vi "LensAndCameraCalibration-GFV.vi"(8 "error in (no error)":errorcluster, 10 "Variant In":variant, 11 "LensCalibrationCtl":T1=enum."Get Calibration") -> (0 "error out":errorcluster, 3 "Variant Out":variant)   [LabVIEW 2013]
doc: "Use this template to build a VI to use as a subVI."
uses:
  LensCalibrationCtlGFV.ctl
  LensCalibrationModel.ctl
  <vilib>/Utility/file.llb/Read From Spreadsheet File (string).vi
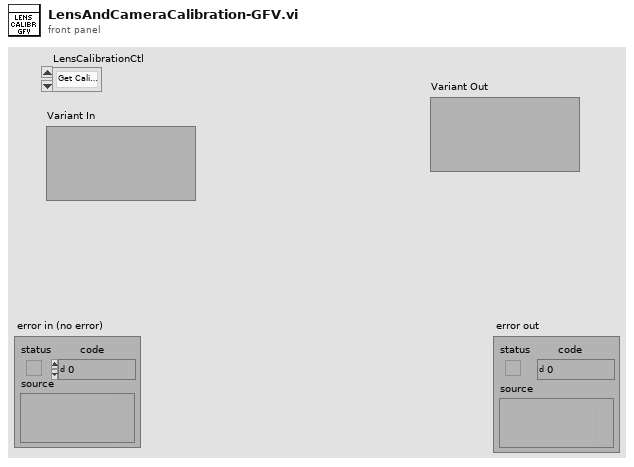
[diagram p1: front panel]
types:
  T1 = typedef "LensCalibrationCtlGFV.ctl" = enum16{"Get MicronPerPixel", "Get Range and PixelsForRange", "Get Mag Names", "Get Calibration", "Read Calibration From File", "Init"}
  T2 = cluster{"MagRingText":u16, "High Resolution":bool}
  T3 = typedef "LensCalibrationModel.ctl" = cluster{"Lens Mag":string, "MicronsPerPixels":dbl, "Scale in microns":i32, "High Resolution":bool}[]
  T4 = cluster{"Lens Mag":string, "MicronsPerPixels":dbl, "Scale in microns":i32, "High Resolution":bool}
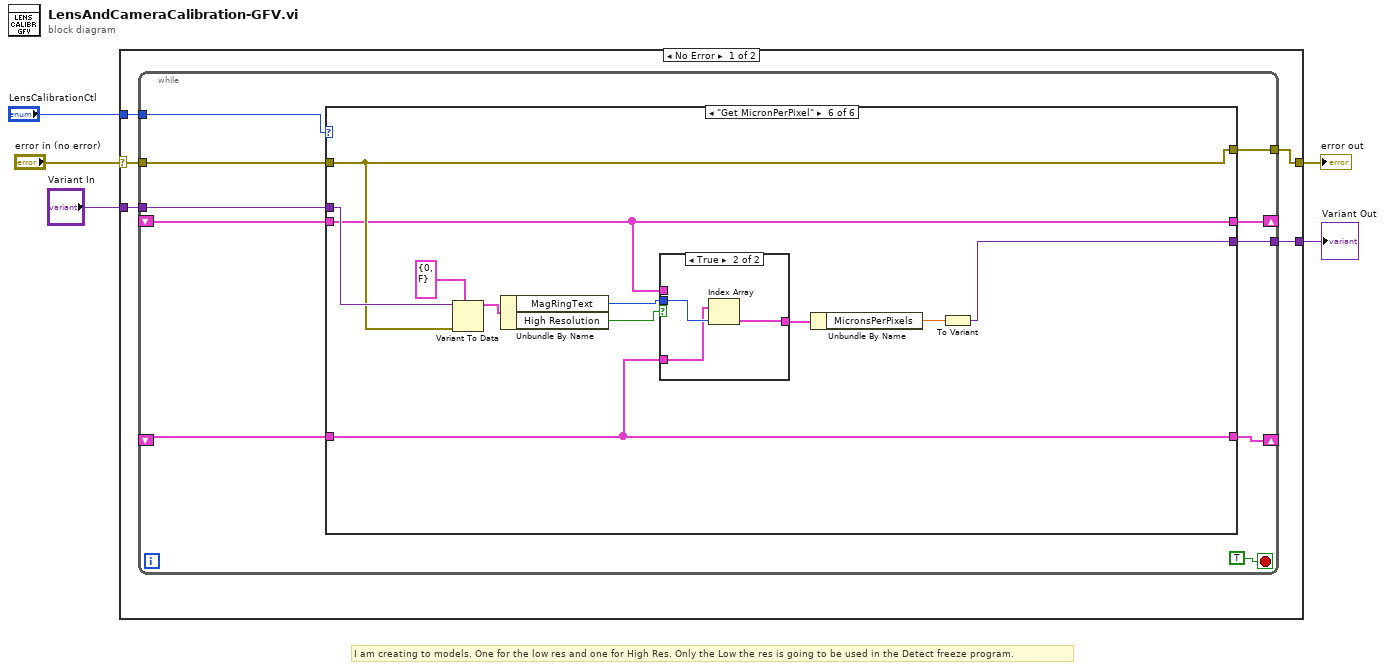
[diagram p0: block diagram]
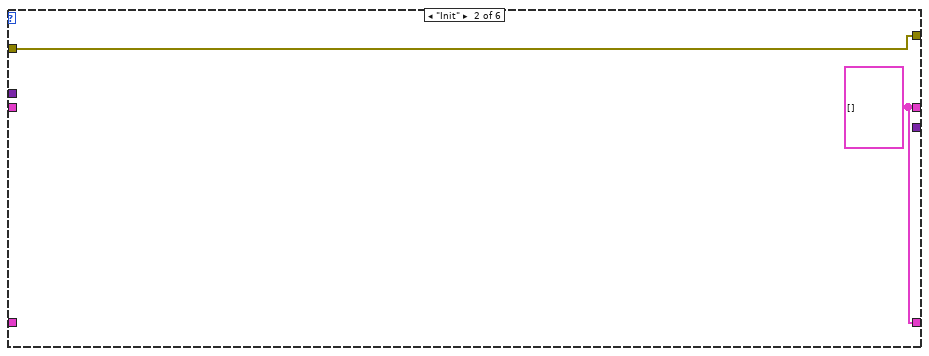
[diagram p3: hidden frame]
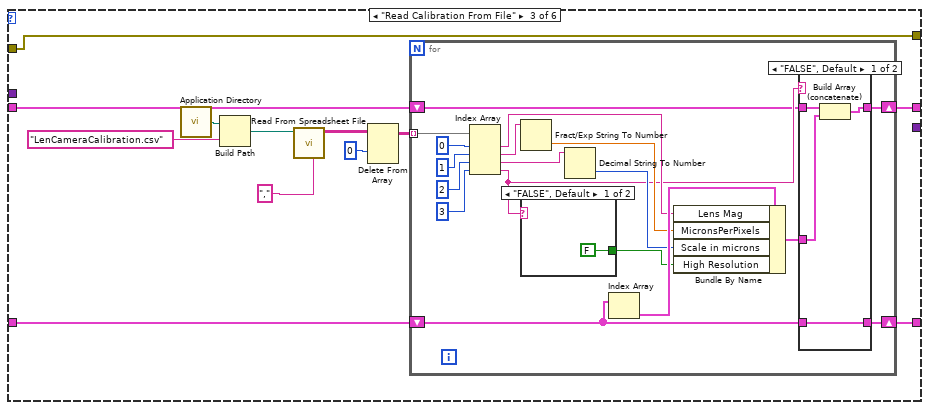
[diagram p4: hidden frame]
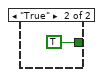
[diagram p5: hidden frame]
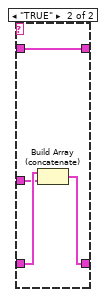
[diagram p6: hidden frame]
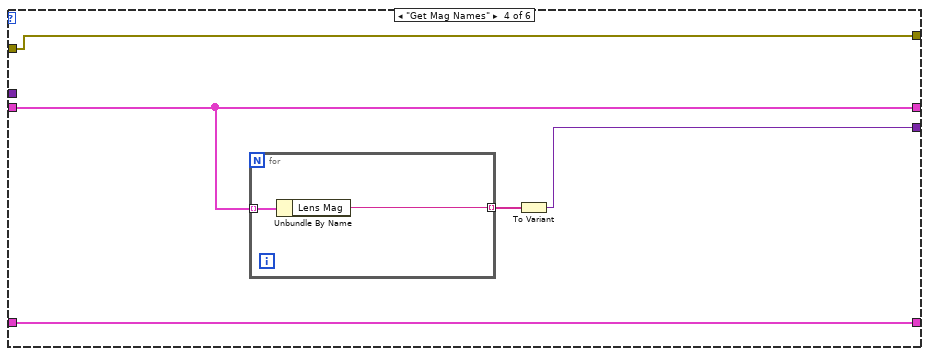
[diagram p7: hidden frame]
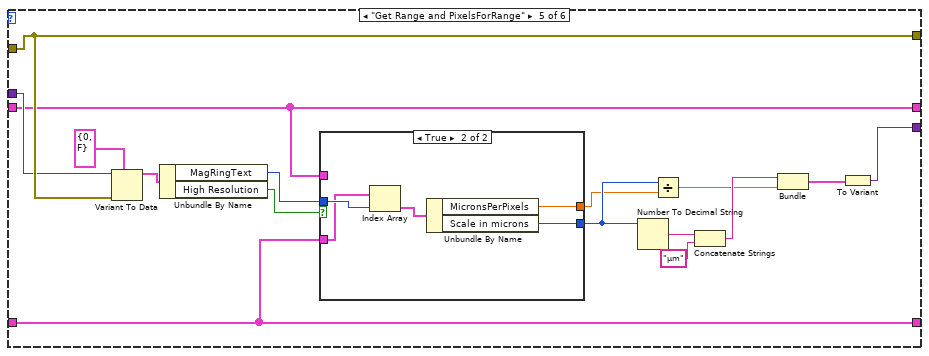
[diagram p8: hidden frame]
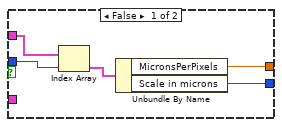
[diagram p9: hidden frame]
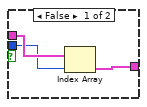
[diagram p10: hidden frame]
diagram:
  # "I am creating to models. One for the low res and one for High Res. Only the Low the res is going to be used in the Detect freeze program."
  n1 = case shown="No Error" "error in (no error)" {
    selector: "error in (no error)" -> [w9 w116]
    tunnel: [w8 w116] -> w4
    tunnel: "LensCalibrationCtl" -> [w10 _]
    tunnel: [w7 _] -> w2
    tunnel: "Variant In" -> [w6 _]
    frame No Error {
      n2 = while {
        tunnel: w10 -> [w19]
        tunnel: w9 -> [w18]
        shift-right: [w14] -> _
        shift-left: _ -> [w15]
        shift-right: [w16] -> _
        shift-left: _ -> [w17]
        tunnel: [w13] -> w8
        tunnel: [w12] -> w7
        tunnel: w6 -> [w11]
        stop <- TRUE stop-if-true
        n3 = case shown="\"Get MicronPerPixel\"" w19 {
          tunnel: w18 -> [w21 w24 w26 w69 w87 w106]
          tunnel: w17 -> [w23 _ w30 w70 w83 w104]
          tunnel: [w23 w25 w29 w70 w83 w104] -> w16
          tunnel: w15 -> [w22 _ w28 w68 w82 w105]
          tunnel: [w22 w25 w27 w68 w82 w105] -> w14
          tunnel: [w21 w24 w26 w69 w87 w106] -> w13
          tunnel: [_ _ _ w66 w77 w99] -> w12
          tunnel: w11 -> [_ _ _ _ w86 w107]
          frame "Get Calibration", Default {
          }
          frame "Init" {
            w25 = T3 [] ("LensLowRes")
          }
          frame "Read Calibration From File" {
            n4 = call <vilib>:"Application Directory.vi"() -> ("Application Directory"=w34:path)
            n5 = Build Path(base path=w34, name or relative path="LenCameraCalibration.csv") -> (appended path=w32:path)
            n6 = call-poly <vilib>:"Read From Spreadsheet File.vi"("delimiter (\\t)"="," ("delimiter (\\t)"), "file path (dialog if empty)"=w32) -> ("all rows"=w36:string[][])  [unwired: 5 in, 4 out]
            n7 = Delete From Array(array=w36, index (row)=0 ("index")) -> (array with subset deleted=w37:string[][])  [unwired: 2 in, 1 out]
            n8 = for {
              tunnel: w37 -> [w55] mode=indexing
              shift-right: [w38] -> w27
              shift-left: w28 -> [w39]
              shift-right: [w45] -> w29
              shift-left: w30 -> [w47]
              n9 = Index Array(array=w55, index #1=0 ("index"), index #2=1 ("index"), index #3=2 ("index"), index #4=3 ("index")) -> (element #1=w44:string, element #2=w50:string, element #3=w49:string, element #4=w41:string)
              n10 = Fract/Exp String To Number(string=w50) -> (number=w43:dbl)  [unwired: 3 in, 1 out]
              n11 = case shown="\"FALSE\", Default" w41 {
                tunnel: [FALSE TRUE] -> w40
                frame "FALSE", Default {
                }
                frame "True" {
                }
              }
              n12 = Decimal String To Number(string=w49) -> (number=w42:i32)  [unwired: 2 in, 1 out]
              n13 = Index Array(array=w47) -> (element=w48:T4)  [unwired: 1 in]
              n14 = Bundle By Name(cluster=w48, "Lens Mag"=w44, "MicronsPerPixels"=w43, "Scale in microns"=w42, "High Resolution"=w40) -> (w46:T4)
              n15 = case shown="\"FALSE\", Default" w41 {
                tunnel: w47 -> [w58 w65]
                tunnel: w46 -> [w60 w64]
                tunnel: [w58 w63] -> w45
                tunnel: w39 -> [w61 w62]
                tunnel: [w59 w62] -> w38
                frame "FALSE", Default {
                  n16 = Build Array (concatenate)(w61, w60) -> (w59:T3)
                }
                frame "TRUE" {
                  n17 = Build Array (concatenate)(w65, w64) -> (w63:T3)
                }
              }
            }
          }
          frame "Get Mag Names" {
            n18 = for {
              tunnel: w68 -> [w72] mode=indexing
              tunnel: [w71] -> w67 mode=indexing
              n19 = Unbundle By Name(w72) -> ("Lens Mag"=w71:string)
            }
            n20 = To Variant(anything=w67) -> (Variant=w66:variant)
          }
          frame "Get Range and PixelsForRange" {
            n21 = Variant To Data(error in=w87, type=T2 {"MagRingText"=0, "High Resolution"=FALSE} ("output cluster"), Variant=w86) -> (data=w85:T2)  [unwired: 1 out]
            n22 = Unbundle By Name(w85) -> ("MagRingText"=w81:u16, "High Resolution"=w84:bool)
            n23 = case shown="True" w84 {
              tunnel: w83 -> [_ w94]
              tunnel: w82 -> [w92 _]
              tunnel: w81 -> [w93 w98]
              tunnel: [w90 w96] -> w74
              tunnel: [w89 w95] -> w75
              frame False {
                n24 = Index Array(array=w92, index=w93) -> (element=w91:T4)
                n25 = Unbundle By Name(w91) -> ("MicronsPerPixels"=w90:dbl, "Scale in microns"=w89:i32)
              }
              frame True {
                n26 = Index Array(array=w94, index=w98) -> (element=w97:T4)
                n27 = Unbundle By Name(w97) -> ("MicronsPerPixels"=w96:dbl, "Scale in microns"=w95:i32)
              }
            }
            n28 = Number To Decimal String(number=w75) -> (decimal integer string=w80:string)  [unwired: 1 in]
            n29 = Divide(x=w75, y=w74) -> (x/y=w73:dbl)
            n30 = Concatenate Strings(w80, "µm" ("string")) -> (w76:string)
            n31 = Bundle(w76, w73) -> (w78:cluster{string, dbl})  [unwired: 1 in]
            n32 = To Variant(anything=w78) -> (Variant=w77:variant)
          }
          frame "Get MicronPerPixel" {
            n33 = Variant To Data(error in=w106, type=T2 {"MagRingText"=0, "High Resolution"=FALSE} ("output cluster"), Variant=w107) -> (data=w108:T2)  [unwired: 1 out]
            n34 = Unbundle By Name(w108) -> ("MagRingText"=w102:u16, "High Resolution"=w103:bool)
            n35 = case shown="True" w103 {
              tunnel: w105 -> [w112 _]
              tunnel: w104 -> [_ w114]
              tunnel: w102 -> [w111 w115]
              tunnel: [w110 w113] -> w101
              frame False {
                n36 = Index Array(array=w112, index=w111) -> (element=w110:T4)
              }
              frame True {
                n37 = Index Array(array=w114, index=w115) -> (element=w113:T4)
              }
            }
            n38 = Unbundle By Name(w101) -> ("MicronsPerPixels"=w100:dbl)
            n39 = To Variant(anything=w100) -> (Variant=w99:variant)
          }
        }
      }
    }
    frame Error {
    }
  }
  "error out" <- w4
  "Variant Out" <- w2
